vi "test visa.vi"() -> ()   [LabVIEW 2012]
uses:
  <vilib>/Instr/_visa.llb/VISA Configure Serial Port (Instr).vi
panel:
  in  "bytes to read":u32
  out "return count write":u32
  out "return count read":u32
  out "read buffer":string
  in  "write buffer":string
  in  "VISA resource name":refnum<visa-resource-name>
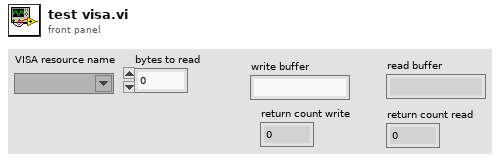
[diagram p1: front panel]
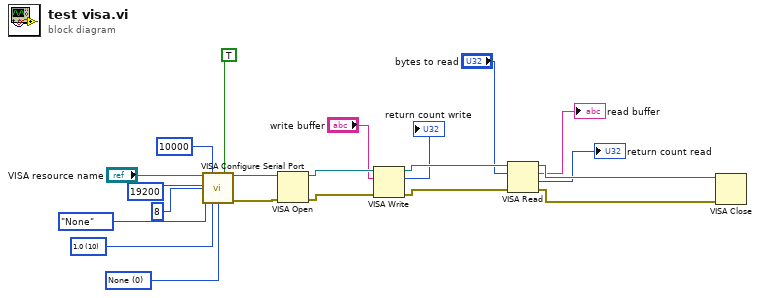
[diagram p0: block diagram]
diagram:
  w15 = u16 0 items=["None", "XON/XOFF", "RTS/CTS", "XON/XOFF & RTS/CTS", "DTR/DSR", "XON/XOFF & DTR/DSR"] ("flow control (0:none)")
  w16 = u16 10 items=["1.0"=10, "1.5"=15, "2.0"=20] ("stop bits (10: 1 bit)")
  n1 = call-poly "VISA Configure Serial Port"("VISA resource name"="VISA resource name", "timeout (10sec)"=u32 10000, "Enable Termination\nChar (T)"=TRUE ("Enable Termination\nChar (T)"), "baud rate (9600)"=u32 19200, "data bits (8)"=u16 8, "parity (0:none)"=enum16{"None", "Odd", "Even", "Mark", "Space"}."None", "stop bits (10: 1 bit)"=w16, "flow control (0:none)"=w15) -> ("VISA resource name out"=w13:refnum<visa-resource-name>, "error out"=w12:errorcluster)  [unwired: 6 in]
  n2 = VISA Open(error in (no error)=w12, VISA resource name=w13) -> (VISA resource name=w11:refnum<visa-resource-name>, error out=w10:errorcluster)  [unwired: 3 in]
  n3 = VISA Write(VISA resource name=w11, write buffer="write buffer", error in (no error)=w10) -> (VISA resource name out=w6:refnum<visa-resource-name>, return count=→"return count write":u32, error out=w8:errorcluster)
  n4 = VISA Read(VISA resource name=w6, byte count="bytes to read", error in (no error)=w8) -> (VISA resource name out=w5:refnum<visa-resource-name>, read buffer=→"read buffer":string, return count=→"return count read":u32, error out=w7:errorcluster)
  n5 = VISA Close(VISA resource name=w5, error in (no error)=w7) -> ()  [unwired: 1 out]
